vi "Mean 4D to 2D.vi"(1 "Array 4D":i32[][][][](array[numeric])) -> (0 "Array 2D":dbl[][](array[numeric]) format="%.2f")   [LabVIEW 2009]
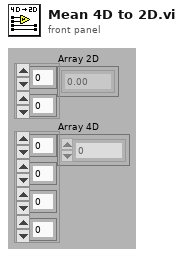
[diagram p1: front panel]
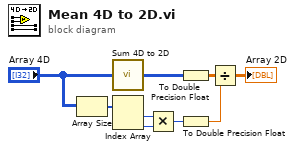
[diagram p0: block diagram]
diagram:
  n1 = Array Size(array="Array 4D") -> (size(s)=w7:i32[])
  n2 = call "Sum 4D to 2D.vi"("Array 4D"="Array 4D") -> ("Array 2D"=w5:i32[][])
  n3 = Index Array(array=w7) -> (element #1=w9:i32, element #2=w8:i32)  [unwired: 2 in]
  n4 = Multiply(x=w9, y=w8) -> (x*y=w2:i32)
  n5 = To Double Precision Float(number=w5) -> (double precision float=w4:dbl[][])
  n6 = To Double Precision Float(number=w2) -> (double precision float=w3:dbl)
  n7 = Divide(x=w4, y=w3) -> (x/y=→"Array 2D":dbl[][])
